vi "5-1 Arrays.vi"() -> ()   [LabVIEW 2014]
doc: "This VI is an exercise in the LabVIEW Core I course.\n\nEnter the number of columns and rows you want generated, then run the VI. This VI generates an array with the number of rows and columns you specify."
panel:
  out "Second Column":dbl[](array[numeric])
  out "Third Row":dbl[](array[numeric])
  out "Array 2":dbl[][](array[numeric])
  out "Intensity Graph":dbl[][](graph)
  out "Array":dbl[][](array[numeric])
  in  "Rows":i32=80
  in  "Columns":i32=80
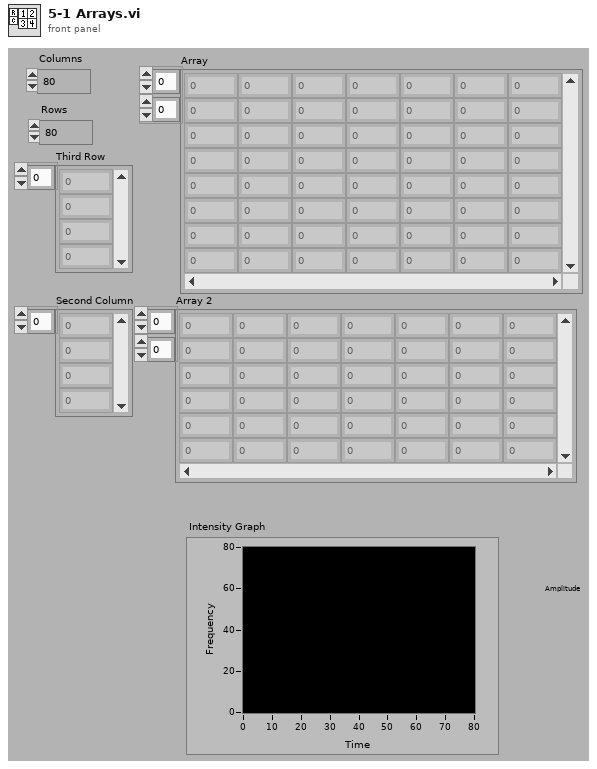
[diagram p1: front panel]
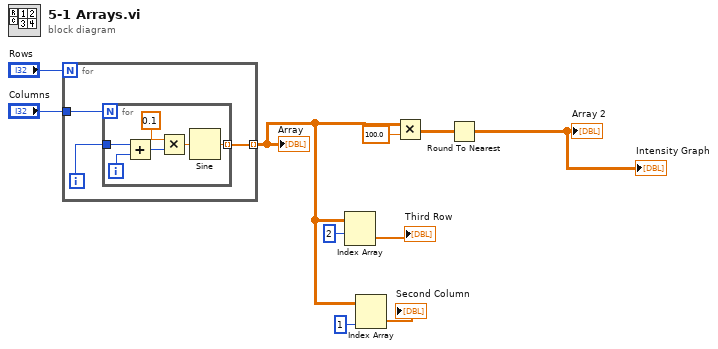
[diagram p0: block diagram]
diagram:
  n1 = for {
    N: "Rows" -> [_]
    tunnel: [w13] -> w5 mode=indexing
    tunnel: "Columns" -> [w12]
    i -> [w11]
    n2 = for {
      N: w12 -> [_]
      tunnel: [w19] -> w13 mode=indexing
      tunnel: w11 -> [w16]
      i -> [w17]
      n3 = Add(x=w16, y=w17) -> (x+y=w18:i32)
      n4 = Multiply(x=0.1, y=w18) -> (x*y=w15:dbl)
      n5 = Sine(x=w15) -> (sin(x)=w19:dbl)
    }
  }
  "Array" <- w5
  n6 = Index Array(array=w5, index (row)=2) -> (element=→"Third Row":dbl[])  [unwired: 1 in]
  n7 = Index Array(array=w5, index (col)=1 ("disabled index (col)")) -> (element=→"Second Column":dbl[])  [unwired: 1 in]
  n8 = Multiply(x=w5, y=100.0) -> (x*y=w6:dbl[][])
  n9 = Round To Nearest(number=w6) -> (nearest integer value=→"Intensity Graph" →"Array 2":dbl[][])
